vi "gps_comparator.vi"() -> ()   [LabVIEW 2019]
panel:
  in  "Tab Control":enum32{"Bemenet", "Gráf"}(tab)
  in  "Stop Button":bool
  in  "Ok button":bool
  out "GPX2":cluster{timestamp[], dbl[]}(graph)
  out "GPX1":cluster{timestamp[], dbl[]}(graph)
  in  "GPX2 path":path
  in  "GPX1 path":path
  in  "Reset":bool
  out "GPX Compare":cluster{dbl[], dbl[]}[](graph)
  in  "Sec":dbl=245.0 format="%#_13g"
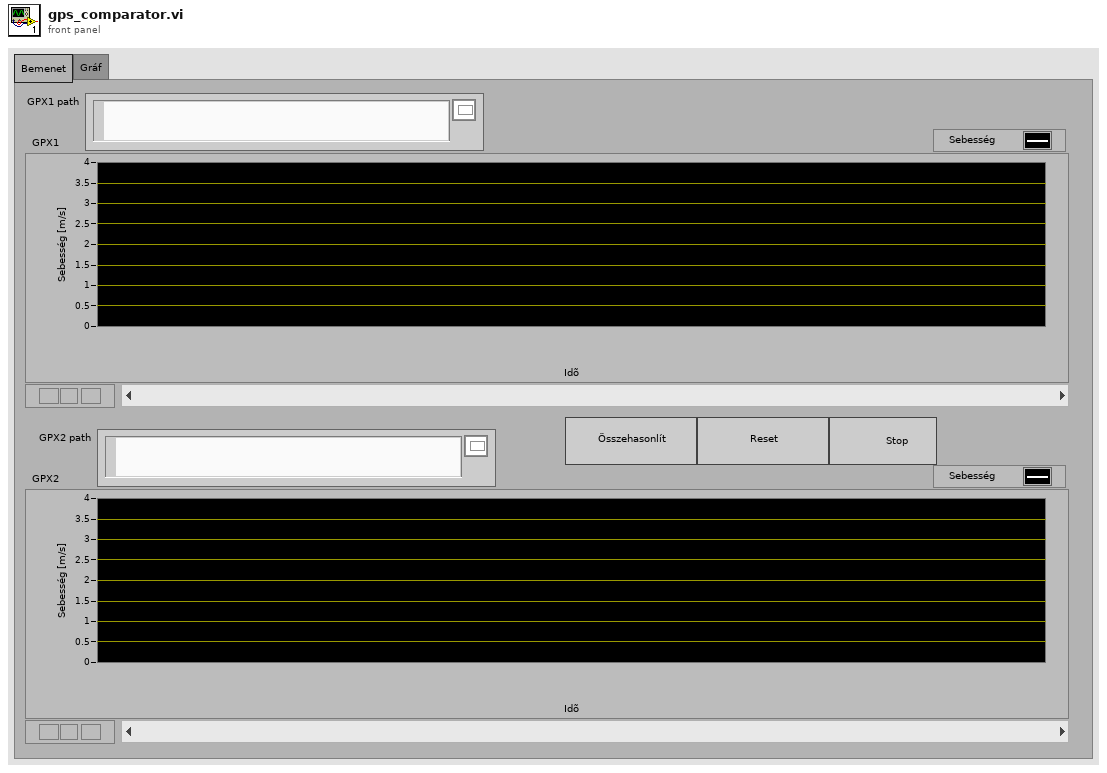
[diagram p1: front panel]
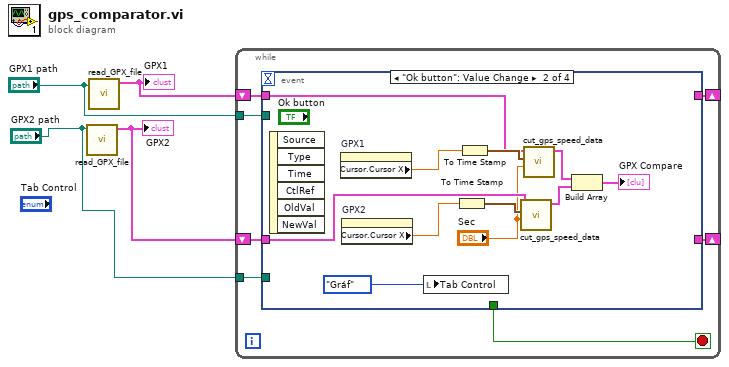
[diagram p0: block diagram]
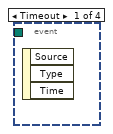
[diagram p2: hidden frame]
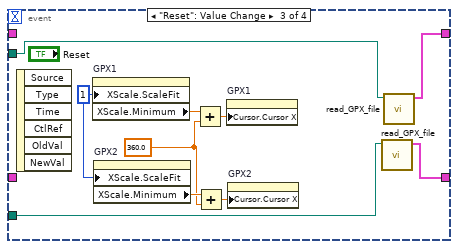
[diagram p3: hidden frame]
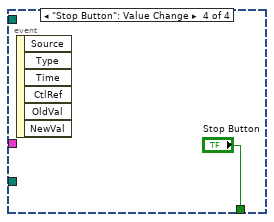
[diagram p4: hidden frame]
diagram:
  n1 = call "read_GPX_file.vi"("GPX File Path"="GPX2 path") -> ("XY Speed data"=w3:cluster{timestamp[], dbl[]})  [unwired: 3 in, 3 out]
  "GPX2" <- w3
  n2 = call "read_GPX_file.vi"("GPX File Path"="GPX1 path") -> ("XY Speed data"=w4:cluster{timestamp[], dbl[]})  [unwired: 3 in, 3 out]
  "GPX1" <- w4
  n3 = while {
    shift-right: [w8] -> _
    shift-left: w4 -> [w10]
    shift-right: [w7] -> _
    shift-left: w3 -> [w9]
    tunnel: "GPX2 path" -> [w6]
    tunnel: "GPX1 path" -> [w5]
    stop <- w11 stop-if-true
    n4 = event shown="[1] \"Ok button\": Value Change" {
      selector: _ -> [_ _ _ _]
      dyn-events: _ -> [_ _ _ _]
      timeout: _ -> [_ _ _ _]
      tunnel: [_ _ _ "Stop Button"] -> w11
      tunnel: w10 -> [_ w14 _ _]
      tunnel: w9 -> [_ w13 _ _]
      tunnel: [_ _ w26 _] -> w8
      tunnel: [_ _ w25 _] -> w7
      tunnel: w6 -> [_ _ w24 _]
      tunnel: w5 -> [_ _ w23 _]
      event Timeout {
        n5 = event-data() -> ()  [unwired: 1 in, 3 out]
      }
      event "Ok button": Value Change {
        n6 = event-data() -> ()  [unwired: 1 in, 6 out]
        n7 = property on="GPX1" class="XYGraph (strict)"() -> ("Cursor.Cursor X"=w19:dbl)  [unwired: 2 in, 2 out]
        n8 = property on="GPX2" class="XYGraph (strict)"() -> ("Cursor.Cursor X"=w16:dbl)  [unwired: 2 in, 2 out]
        n9 = local write "Tab Control"(enum32{"Bemenet", "Gráf"}."Gráf" ("Tab Control")) -> ()
        n10 = To Time Stamp(1:w16) -> (0:w18:timestamp)
        n11 = To Time Stamp(1:w19) -> (0:w20:timestamp)
        n12 = call "cut_gps_speed_data.vi"("Sec"="Sec", "Start Time"=w18, "timestamp gps speed data"=w13) -> ("XY gps speed data"=w17:cluster{dbl[], dbl[]})  [unwired: 8 in]
        n13 = call "cut_gps_speed_data.vi"("Sec"="Sec", "Start Time"=w20, "timestamp gps speed data"=w14) -> ("XY gps speed data"=w21:cluster{dbl[], dbl[]})  [unwired: 8 in]
        n14 = Build Array(w21, w17) -> (→"GPX Compare":cluster{dbl[], dbl[]}[])
      }
      event "Reset": Value Change {
        w28 = 360.0 ("y")
        w27 = u8 1 ("X Scale.Scale Fit")
        n15 = event-data() -> ()  [unwired: 1 in, 6 out]
        n16 = property on="GPX1" class="XYGraph (strict)"("XScale.ScaleFit"=w27) -> ("XScale.Minimum"=w32:dbl)  [unwired: 2 in, 2 out]
        n17 = property on="GPX2" class="XYGraph (strict)"("XScale.ScaleFit"=w27) -> ("XScale.Minimum"=w29:dbl)  [unwired: 2 in, 2 out]
        n18 = Add(x=w32, y=w28) -> (x+y=w31:dbl)
        n19 = Add(x=w29, y=w28) -> (x+y=w30:dbl)
        n20 = property on="GPX1" class="XYGraph (strict)"("Cursor.Cursor X"=w31) -> ()  [unwired: 2 in, 2 out]
        n21 = property on="GPX2" class="XYGraph (strict)"("Cursor.Cursor X"=w30) -> ()  [unwired: 2 in, 2 out]
        n22 = call "read_GPX_file.vi"("GPX File Path"=w24) -> ("XY Speed data"=w25:cluster{timestamp[], dbl[]})  [unwired: 3 in, 3 out]
        n23 = call "read_GPX_file.vi"("GPX File Path"=w23) -> ("XY Speed data"=w26:cluster{timestamp[], dbl[]})  [unwired: 3 in, 3 out]
      }
      event "Stop Button": Value Change {
        n24 = event-data() -> ()  [unwired: 1 in, 6 out]
      }
    }
  }
